vi "De-embed S-parameters - execute.vi"(4 "Truncate index":i32, 5 "Right info":T1, 6 "Truncate files":bool, 7 "Left info":T1, 8 "error in (no error)":errorcluster, 9 "Ignore lowest freq":bool caption="Ignore lowest frequency point (ISD discards it)", 10 "Horizontal Progress Bar":refnum<vi>, 11 "DUT+Fixture":path) -> (0 "error out":errorcluster)   [LabVIEW 2020]
uses:
  <vilib>/addons/HF Network Analysis/Support VIs/Read SnP File (SnP).vi
  <vilib>/addons/HF Network Analysis/NI_HFNetworkAnalysis.lvlib
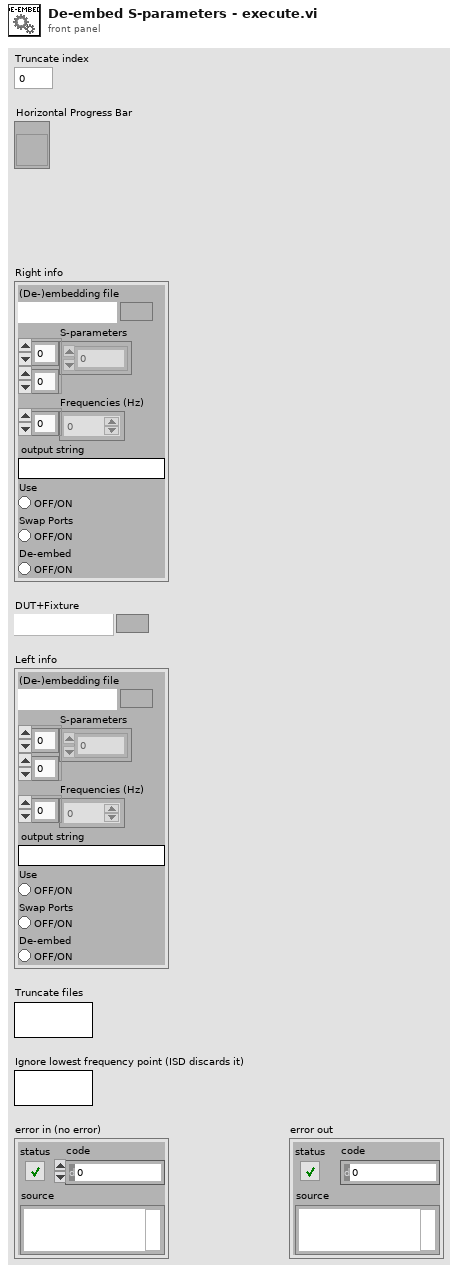
[diagram p1: front panel]
types:
  T1 = cluster{"(De-)embedding file":path, "S-parameters":cdb[][], "Frequencies (Hz)":dbl[], "output string":string, "Use":bool, "Swap Ports":bool, "De-embed":bool}
  T2 = enum16{"Check", "Read left", "Read right", "De-embed", "Exit"}
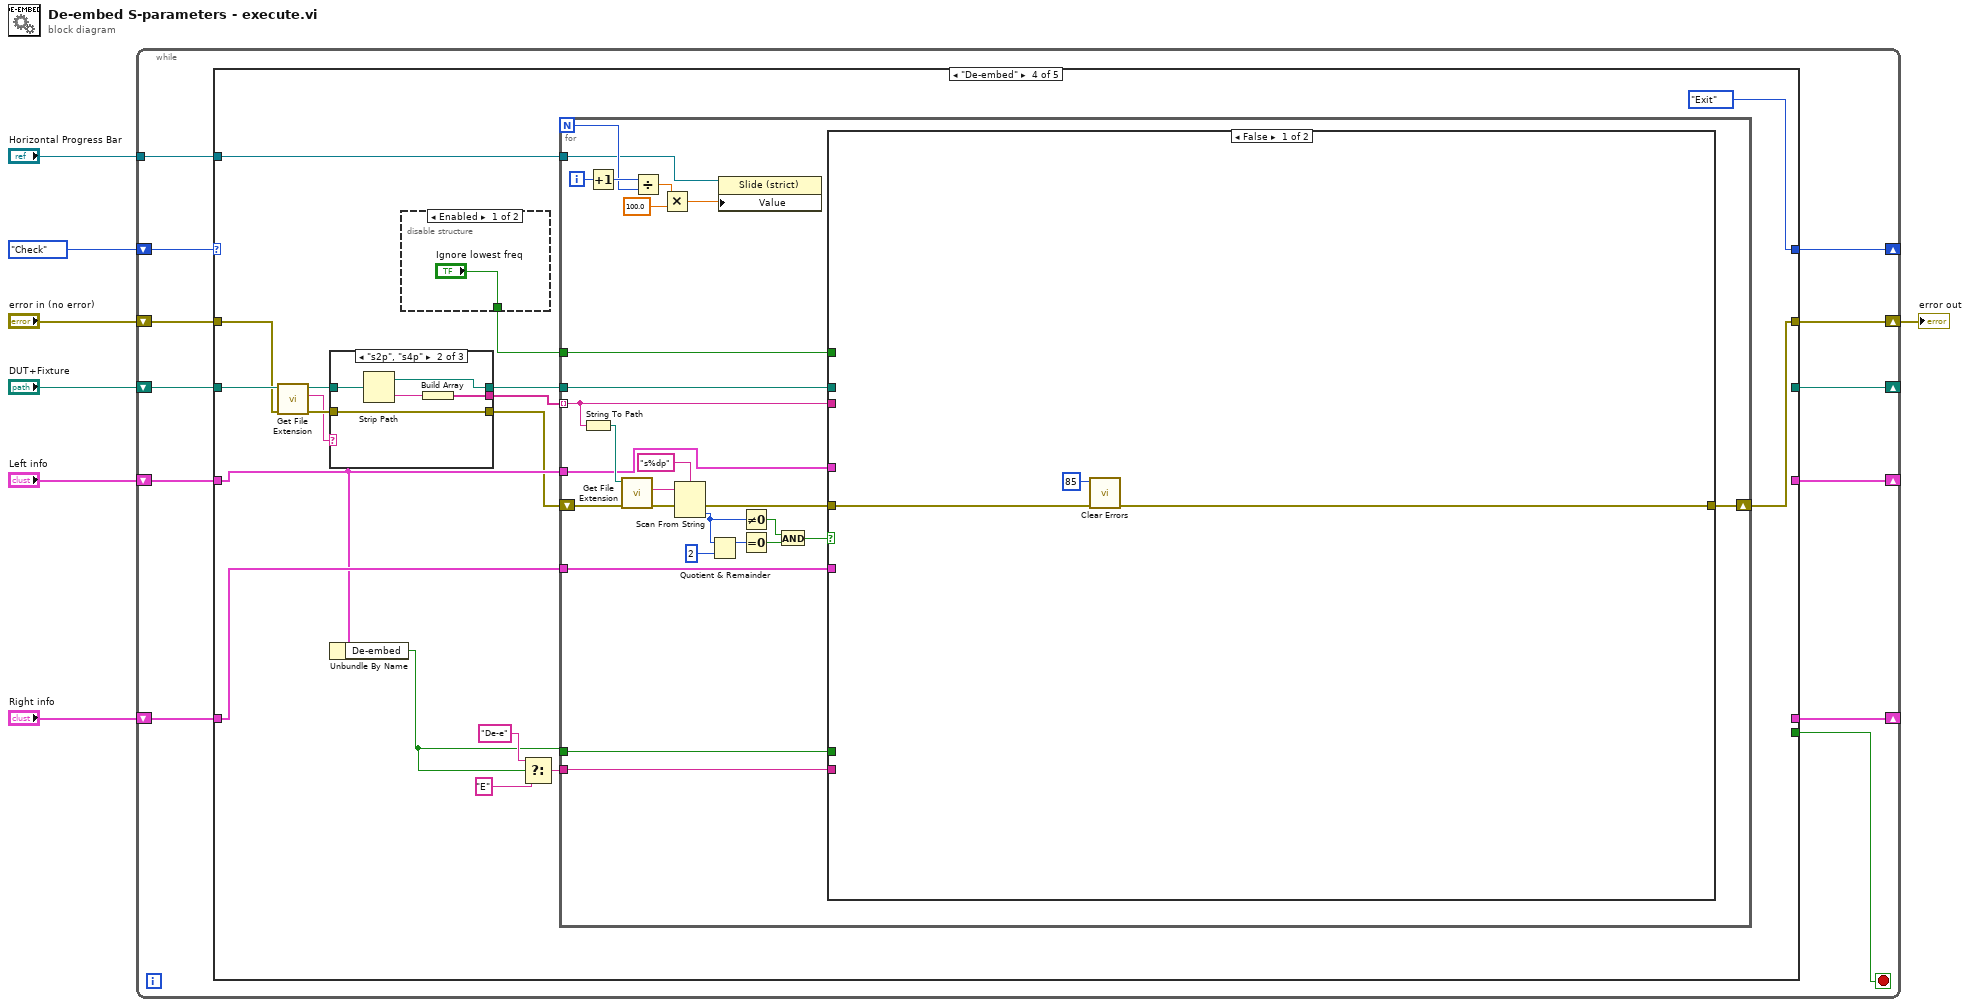
[diagram p0: block diagram]
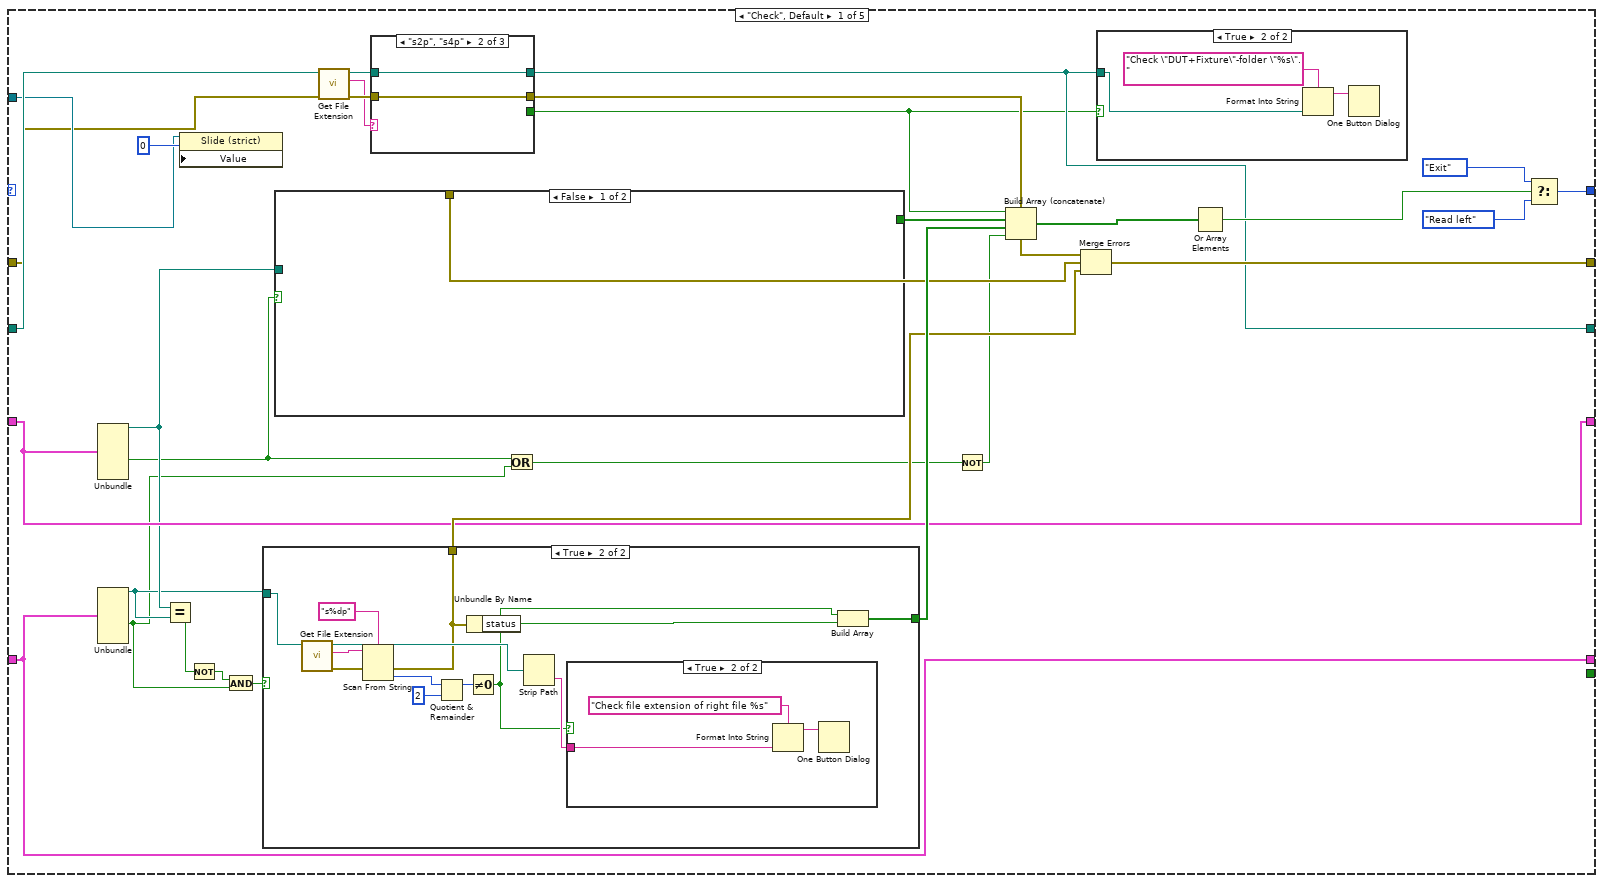
[diagram p2: hidden frame]
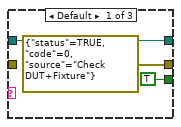
[diagram p3: hidden frame]
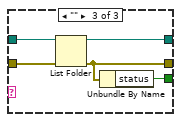
[diagram p4: hidden frame]
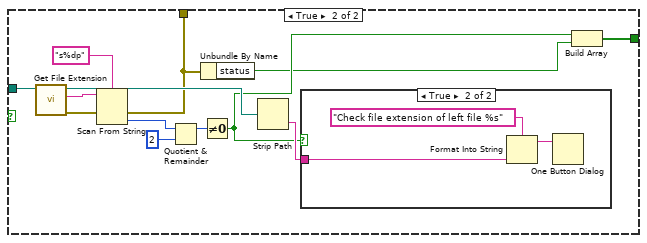
[diagram p6: hidden frame]
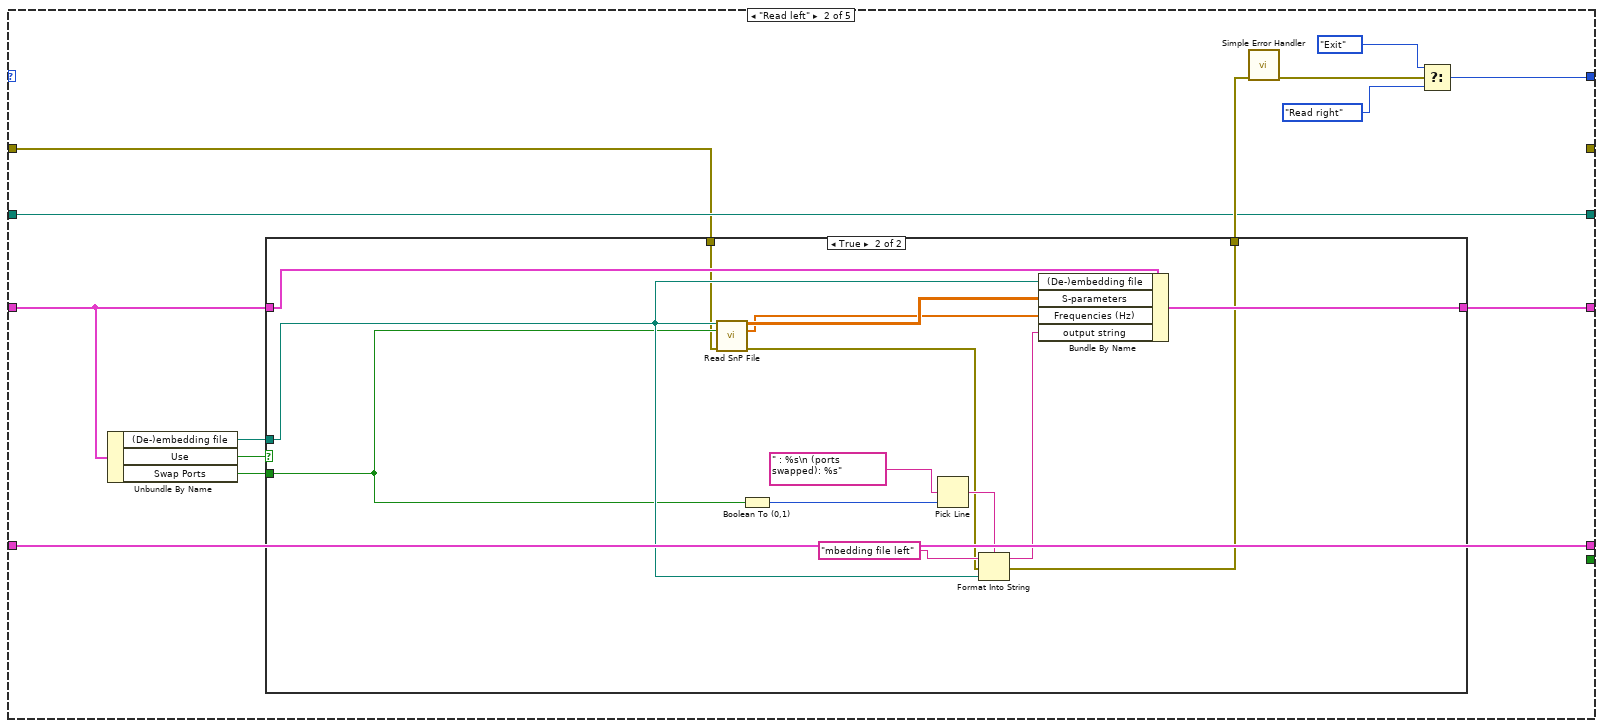
[diagram p10: hidden frame]
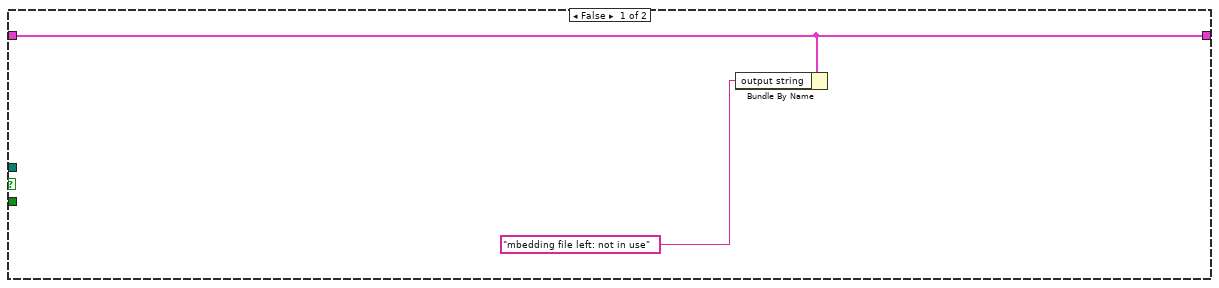
[diagram p11: hidden frame]
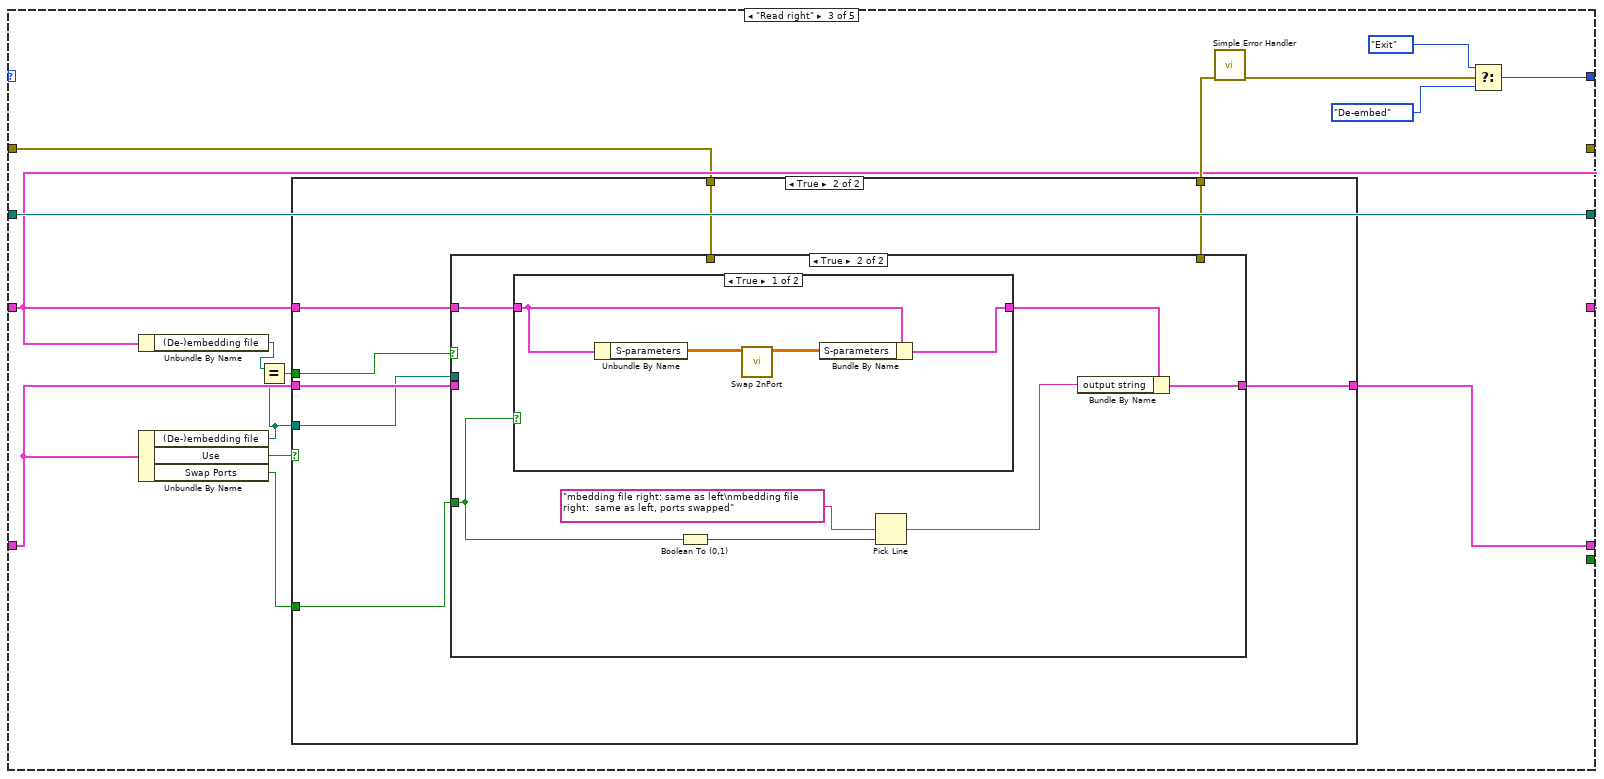
[diagram p12: hidden frame]
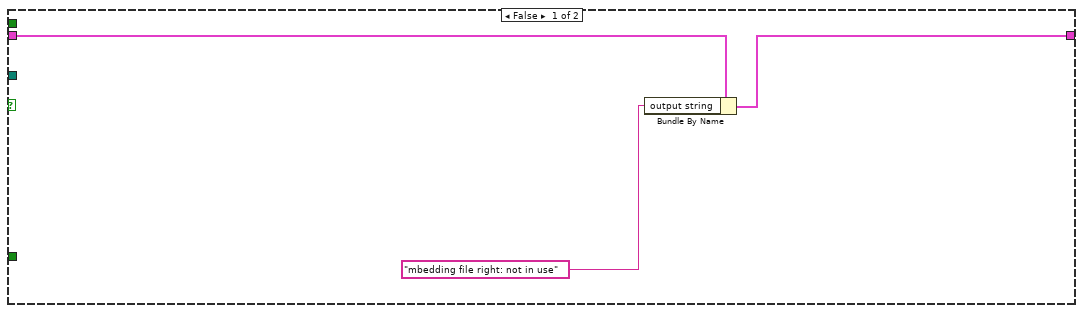
[diagram p13: hidden frame]
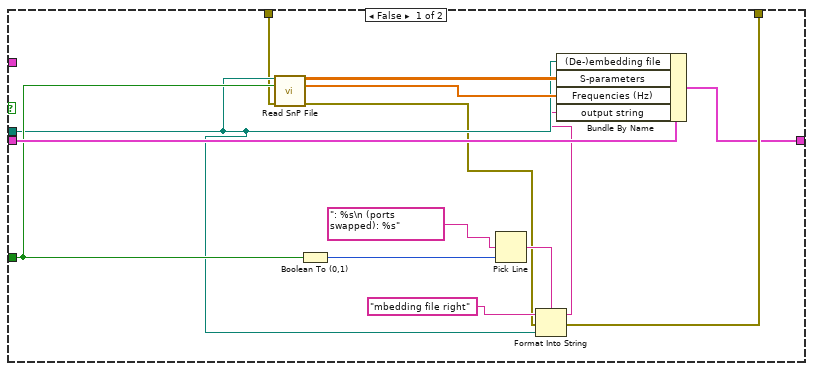
[diagram p14: hidden frame]
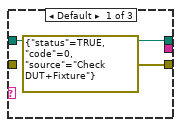
[diagram p17: hidden frame]
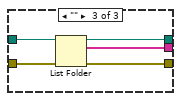
[diagram p18: hidden frame]
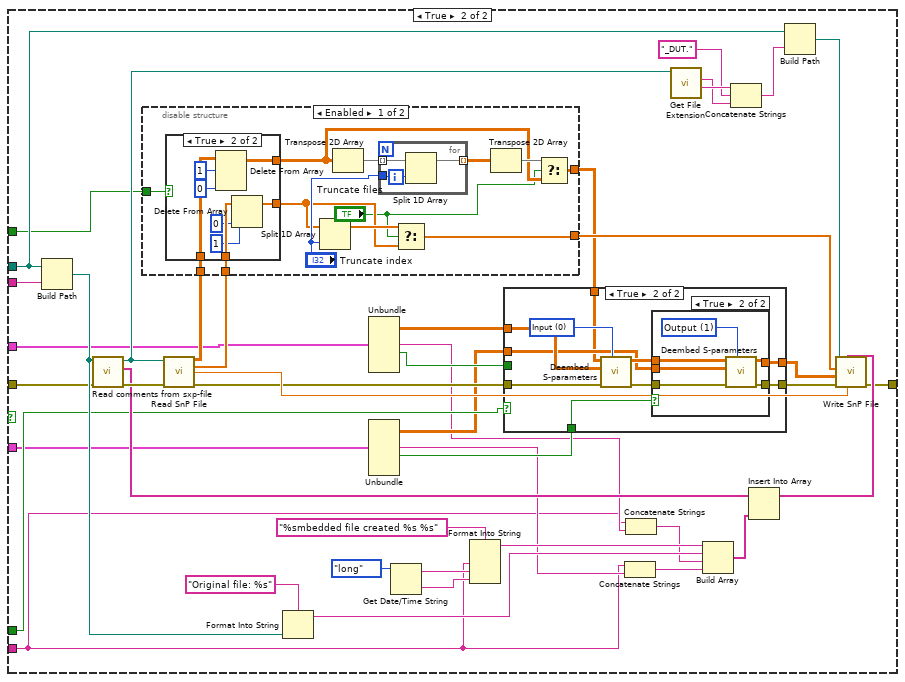
[diagram p19: hidden frame]
diagram:
  n1 = while {
    shift-right: [w16] -> _
    shift-left: "DUT+Fixture" -> [w18]
    shift-right: [w15] -> _
    shift-left: T2."Check" -> [w19]
    shift-right: [w14] -> _
    shift-left: "Left info" -> [w12]
    shift-right: [w13] -> _
    shift-left: "Right info" -> [w11]
    shift-right: [w10] -> w3
    shift-left: "error in (no error)" -> [w9]
    tunnel: "Horizontal Progress Bar" -> [w8]
    stop <- w17 stop-if-true
    n2 = case shown="\"De-embed\"" w19 {
      tunnel: w11 -> [w35 w103 w132 w189 w352]
      tunnel: w12 -> [w36 w100 w130 w188 w353]
      tunnel: w18 -> [w31 w102 w134 w182 _]
      tunnel: [_ _ _ _ TRUE] -> w17
      tunnel: [w22 w102 w134 _ path "" ("path out")] -> w16
      tunnel: [w46 w106 w137 T2."Exit" T2."Check"] -> w15
      tunnel: [w36 w101 w130 _ w353] -> w14
      tunnel: [w35 w103 w133 _ w352] -> w13
      tunnel: [w37 _ _ w179 w351] -> w10
      tunnel: w9 -> [w21 w96 w125 w178 w351]
      tunnel: w8 -> [w27 _ _ w186 _]
      frame "Check", Default {
        n3 = Unbundle(w36) -> ("(De-)embedding file"=w34:path, "Use"=w26:bool)  [unwired: 5 out]
        n4 = Unbundle(w35) -> ("(De-)embedding file"=w33:path, "Use"=w25:bool)  [unwired: 5 out]
        n5 = Equal?(x=w34, y=w33) -> (x = y?=w32:bool)
        n6 = property class="Slide (strict)"(reference=w27, "Value"=u8 0 ("Horizontal Progress Bar")) -> ()  [unwired: 1 in, 2 out]
        n7 = Not(x=w32) -> (.not. x?=w43:bool)
        n8 = And(x=w43, y=w25) -> (x .and. y?=w42:bool)
        n9 = case shown="True" w42 {
          tunnel: w33 -> [_ w85]
          tunnel: [_ w81] -> w44
          tunnel: [_ w80] -> w38
          frame False {
          }
          frame True {
            n10 = call <vilib>:"Get File Extension.vi"("file"=w85) -> ("error out"=w88:errorcluster, "lowercase file extension"=w86:string, "dup file"=w84:path)  [unwired: 6 in, 2 out]
            n11 = Scan From String(format string="s%dp", input string=w86, error in=w88) -> (error out=w80:errorcluster, output 1=w91:i32)  [unwired: 2 in, 2 out]
            n12 = Quotient & Remainder(x=w91, y=2) -> (x-y*floor(x/y)=w90:i32)  [unwired: 1 out]
            n13 = Unbundle By Name(w80) -> ("status"=w82:bool)
            n14 = Not Equal To 0?(x=w90) -> (x != 0?=w83:bool)
            n15 = Strip Path(path=w84) -> (name=w92:string)  [unwired: 1 out]
            n16 = case shown="True" w83 {
              tunnel: w92 -> [_ w93]
              frame False {
              }
              frame True {
                n17 = Format Into String(format string="Check file extension of right file %s", w93) -> (resulting string=w94:string)  [unwired: 2 in, 1 out]
                n18 = One Button Dialog(message=w94) -> ()  [unwired: 1 in, 1 out]
              }
            }
            n19 = Build Array(w83, w82) -> (w81:bool[])
          }
        }
        n20 = case shown="False" w26 {
          tunnel: [_ w65] -> w45
          tunnel: w34 -> [_ w69]
          tunnel: [_ w64] -> w39
          frame False {
          }
          frame True {
            n21 = call <vilib>:"Get File Extension.vi"("file"=w69) -> ("error out"=w74:errorcluster, "lowercase file extension"=w76:string, "dup file"=w68:path)  [unwired: 6 in, 2 out]
            n22 = Scan From String(format string="s%dp", input string=w76, error in=w74) -> (error out=w64:errorcluster, output 1=w71:i32)  [unwired: 2 in, 2 out]
            n23 = Quotient & Remainder(x=w71, y=2) -> (x-y*floor(x/y)=w72:i32)  [unwired: 1 out]
            n24 = Unbundle By Name(w64) -> ("status"=w66:bool)
            n25 = Not Equal To 0?(x=w72) -> (x != 0?=w67:bool)
            n26 = Strip Path(path=w68) -> (name=w70:string)  [unwired: 1 out]
            n27 = case shown="True" w67 {
              tunnel: w70 -> [_ w77]
              frame False {
              }
              frame True {
                n28 = Format Into String(format string="Check file extension of left file %s", w77) -> (resulting string=w78:string)  [unwired: 2 in, 1 out]
                n29 = One Button Dialog(message=w78) -> ()  [unwired: 1 in, 1 out]
              }
            }
            n30 = Build Array(w67, w66) -> (w65:bool[])
          }
        }
        n31 = call <vilib>:"Get File Extension.vi"("error in (no error)"=w21, "file"=w31) -> ("error out"=w29:errorcluster, "lowercase file extension"=w28:string, "dup file"=w30:path)  [unwired: 5 in, 2 out]
        n32 = case shown="\"s2p\", \"s4p\"" w28 {
          tunnel: [errorcluster {"status"=TRUE, "code"=0, "source"="Check DUT+Fixture"} ("error out") w55 w60] -> w40
          tunnel: [w53 w54 w59] -> w22
          tunnel: w30 -> [w53 w54 w58]
          tunnel: w29 -> [_ w55 w57]
          tunnel: [TRUE ("status") _ w56] -> w20
          frame Default {
          }
          frame "s2p", "s4p" {
          }
          frame "" {
            n33 = List Folder(path=w58, error in=w57) -> (path out=w59:path, error out=w60:errorcluster)  [unwired: 2 in, 2 out]
            n34 = Unbundle By Name(w60) -> ("status"=w56:bool)
          }
        }
        n35 = Or(x=w26, y=w25) -> (x .or. y?=w24:bool)
        n36 = Not(x=w24) -> (.not. x?=w23:bool)
        n37 = Build Array (concatenate)(w20, w45, w44, w23) -> (w50:bool[])
        n38 = Merge Errors(w40, w39, w38) -> (w37:errorcluster)
        n39 = case shown="True" w20 {
          tunnel: w22 -> [_ w61]
          frame False {
          }
          frame True {
            n40 = Format Into String(format string="Check \"DUT+Fixture\"-folder \"%s\".", w61) -> (resulting string=w62:string)  [unwired: 2 in, 1 out]
            n41 = One Button Dialog(message=w62) -> ()  [unwired: 1 in, 1 out]
          }
        }
        n42 = Or Array Elements(Boolean array=w50) -> (logical OR=w47:bool)
        n43 = Select(t=T2."Exit", s=w47, f=T2."Read left") -> (s? t:f=w46:T2)
      }
      frame "Read left" {
        n44 = Unbundle By Name(w100) -> ("(De-)embedding file"=w98:path, "Use"=w99:bool, "Swap Ports"=w97:bool)
        n45 = case shown="True" w99 {
          tunnel: [_ w113] -> w105
          tunnel: [w110 w120] -> w101
          tunnel: w100 -> [w110 w119]
          tunnel: w98 -> [_ w117]
          tunnel: w97 -> [_ w112]
          tunnel: w96 -> [_ w111]
          frame False {
            n46 = Bundle By Name(cluster=w110, "output string"="mbedding file left: not in use" ("format string")) -> ()  [unwired: 1 out]
          }
          frame True {
            n47 = call-poly <vilib>:"Read SnP File.vi"("SnP File Path"=w117, "Swap Ports (False)"=w112, "Error In"=w111) -> ("S-parameters"=w124:cdb[][], "Frequencies (Hz)"=w123:dbl[], "Error Out"=w114:errorcluster)  [unwired: 9 in, 1 out]
            n48 = Boolean To (0,1)(Boolean=w112) -> (0, 1=w122:i16)
            n49 = Pick Line(multi-line string=" : %s\n (ports swapped): %s" ("format string"), line index=w122) -> (output string=w116:string)  [unwired: 1 in]
            n50 = Format Into String(format string=w116, initial string="mbedding file left" ("format string"), error in=w114, w117) -> (resulting string=w115:string, error out=w113:errorcluster)
            n51 = Bundle By Name(cluster=w119, "(De-)embedding file"=w117, "S-parameters"=w124, "Frequencies (Hz)"=w123, "output string"=w115) -> (w120:T1)
          }
        }
        n52 = call <vilib>:"Simple Error Handler.vi"("error in (no error)"=w105) -> ("error out"=w104:errorcluster)  [unwired: 4 in, 4 out]
        n53 = Select(t=T2."Exit", s=w104, f=T2."Read right") -> (s? t:f=w106:T2)
      }
      frame "Read right" {
        n54 = Unbundle By Name(w130) -> ("(De-)embedding file"=w129:path)
        n55 = Unbundle By Name(w132) -> ("(De-)embedding file"=w128:path, "Use"=w131:bool, "Swap Ports"=w126:bool)
        n56 = Equal?(x=w129, y=w128) -> (x = y?=w127:bool)
        n57 = case shown="True" w131 {
          tunnel: [_ w150] -> w136
          tunnel: [w140 w143] -> w133
          tunnel: w130 -> [_ w144]
          tunnel: w132 -> [w141 w149]
          tunnel: w128 -> [_ w148]
          tunnel: w127 -> [_ w147]
          tunnel: w126 -> [_ w146]
          tunnel: w125 -> [_ w145]
          frame False {
            n58 = Bundle By Name(cluster=w141, "output string"="mbedding file right: not in use" ("format string")) -> (w140:T1)
          }
          frame True {
            n59 = case shown="True" w147 {
              tunnel: [w154 _] -> w150
              tunnel: w148 -> [w158 _]
              tunnel: w149 -> [w162 _]
              tunnel: w146 -> [w161 w167]
              tunnel: w145 -> [w152 _]
              tunnel: w144 -> [_ w166]
              tunnel: [w151 w168] -> w143
              frame False {
                n60 = call-poly <vilib>:"Read SnP File.vi"("SnP File Path"=w158, "Swap Ports (False)"=w161, "Error In"=w152) -> ("S-parameters"=w164:cdb[][], "Frequencies (Hz)"=w163:dbl[], "Error Out"=w155:errorcluster)  [unwired: 9 in, 1 out]
                n61 = Boolean To (0,1)(Boolean=w161) -> (0, 1=w153:i16)
                n62 = Pick Line(multi-line string=": %s\n (ports swapped): %s" ("format string"), line index=w153) -> (output string=w157:string)  [unwired: 1 in]
                n63 = Format Into String(format string=w157, initial string="mbedding file right" ("format string"), error in=w155, w158) -> (resulting string=w156:string, error out=w154:errorcluster)
                n64 = Bundle By Name(cluster=w162, "(De-)embedding file"=w158, "S-parameters"=w164, "Frequencies (Hz)"=w163, "output string"=w156) -> (w151:T1)
              }
              frame True {
                n65 = case shown="True" w167 {
                  tunnel: w166 -> [w174 w176]
                  tunnel: [w175 w176] -> w165
                  frame True {
                    n66 = Unbundle By Name(w174) -> ("S-parameters"=w173:cdb[][])
                    n67 = call <vilib>:"Swap 2nPort.vi"("Parameters In (2D)"=w173) -> ("Parameters Out (2D)"=w172:cdb[][])  [unwired: 9 in, 1 out]
                    n68 = Bundle By Name(cluster=w174, "S-parameters"=w172) -> (w175:T1)
                  }
                  frame False {
                  }
                }
                n69 = Boolean To (0,1)(Boolean=w167) -> (0, 1=w171:i16)
                n70 = Pick Line(multi-line string="mbedding file right: same as left\nmbedding file right:  same as left, ports swapped" ("format string"), line index=w171) -> (output string=w169:string)  [unwired: 1 in]
                n71 = Bundle By Name(cluster=w165, "output string"=w169) -> (w168:T1)
              }
            }
          }
        }
        n72 = call <vilib>:"Simple Error Handler.vi"("error in (no error)"=w136) -> ("error out"=w135:errorcluster)  [unwired: 4 in, 4 out]
        n73 = Select(t=T2."Exit", s=w135, f=T2."De-embed") -> (s? t:f=w137:T2)
      }
      frame "De-embed" {
        n74 = call <vilib>:"Get File Extension.vi"("error in (no error)"=w178, "file"=w182) -> ("error out"=w184:errorcluster, "lowercase file extension"=w183:string, "dup file"=w185:path)  [unwired: 5 in, 2 out]
        n75 = case shown="\"s2p\", \"s4p\"" w183 {
          tunnel: [errorcluster {"status"=TRUE, "code"=0, "source"="Check DUT+Fixture"} ("error out") w202 w207] -> w177
          tunnel: [w197 w200 w206] -> w181
          tunnel: w185 -> [w197 w201 w205]
          tunnel: w184 -> [_ w202 w204]
          tunnel: [_ w198 w203] -> w180
          frame Default {
          }
          frame "s2p", "s4p" {
            n76 = Strip Path(path=w201) -> (stripped path=w200:path, name=w199:string)
            n77 = Build Array(w199) -> (w198:string[])
          }
          frame "" {
            n78 = List Folder(path=w205, error in=w204) -> (path out=w206:path, filenames=w203:string[], error out=w207:errorcluster)  [unwired: 2 in, 1 out]
          }
        }
        n79 = Unbundle By Name(w188) -> ("De-embed"=w187:bool)
        n80 = disable-structure shown="Enabled" {
          disable-tunnel: ["Ignore lowest freq" _] -> w194
          frame Enabled {
          }
          frame Disabled {
          }
        }
        n81 = Select(t="De-e" ("format string"), s=w187, f="E" ("format string")) -> (s? t:f=w191:string)
        n82 = for {
          N -> [w212]
          tunnel: w181 -> [w234]
          tunnel: w180 -> [w233] mode=indexing
          tunnel: w194 -> [w229]
          tunnel: w191 -> [w228]
          tunnel: w187 -> [w227]
          tunnel: w188 -> [w216]
          tunnel: w189 -> [w215]
          tunnel: w186 -> [w211]
          shift-right: [w209] -> w179
          shift-left: w177 -> [w208]
          i -> [w231]
          n83 = String To Path(string=w233) -> (path=w232:path)
          n84 = Increment(x=w231) -> (x+1=w230:i32)
          n85 = call <vilib>:"Get File Extension.vi"("error in (no error)"=w208, "file"=w232) -> ("error out"=w226:errorcluster, "lowercase file extension"=w224:string)  [unwired: 5 in, 3 out]
          n86 = Divide(x=w230, y=w212) -> (x/y=w214:dbl)
          n87 = Multiply(x=w214, y=100.0) -> (x*y=w210:dbl)
          n88 = Scan From String(format string="s%dp", input string=w224, error in=w226) -> (error out=w225:errorcluster, output 1=w218:i32)  [unwired: 2 in, 2 out]
          n89 = Quotient & Remainder(x=w218, y=2) -> (x-y*floor(x/y)=w222:i32)  [unwired: 1 out]
          n90 = property class="Slide (strict)"(reference=w211, "Value"=w210) -> ()  [unwired: 1 in, 2 out]
          n91 = Not Equal To 0?(x=w218) -> (x != 0?=w217:bool)
          n92 = Equal To 0?(x=w222) -> (x = 0?=w220:bool)
          n93 = And(x=w217, y=w220) -> (x .and. y?=w219:bool)
          n94 = case shown="False" w219 {
            tunnel: w233 -> [_ w272]
            tunnel: w234 -> [_ w261]
            tunnel: w225 -> [w237 w258]
            tunnel: w229 -> [_ w253]
            tunnel: w228 -> [_ w239]
            tunnel: w227 -> [_ w250]
            tunnel: w216 -> [_ w249]
            tunnel: w215 -> [_ w246]
            tunnel: [w236 w238] -> w209
            frame False {
              n95 = call <vilib>:"Clear Errors.vi"("error in (no error)"=w237, "specific error code to clear (0: all)"=85) -> ("error out"=w236:errorcluster)  [unwired: 4 in, 1 out]
            }
            frame True {
              n96 = Build Path(base path=w261, name or relative path=w272) -> (appended path=w260:path)
              n97 = call "Read comments from sxp-file.vi"("error in (no error)"=w258, "file path"=w260) -> ("error out"=w257:errorcluster, "Comment lines"=w254:string[], "file path out"=w259:path)  [unwired: 7 in]
              n98 = call-poly <vilib>:"Read SnP File.vi"("SnP File Path"=w259, "Error In"=w257) -> ("S-parameters"=w264:cdb[][], "Frequencies (Hz)"=w263:dbl[], "Z0 (Ohm)"=w280:cdb, "Error Out"=w262:errorcluster)  [unwired: 10 in]
              n99 = disable-structure shown="Enabled" {
                disable-tunnel: w264 -> [w293 w308]
                disable-tunnel: w263 -> [w292 w307]
                disable-tunnel: w253 -> [w291 _]
                disable-tunnel: [w285 w307] -> w252
                disable-tunnel: [w283 w308] -> w251
                frame Enabled {
                  n100 = case shown="True" w291 {
                    tunnel: w293 -> [w297 w306]
                    tunnel: [w297 w305] -> w282
                    tunnel: w292 -> [w298 w304]
                    tunnel: [w298 w303] -> w286
                    frame False {
                    }
                    frame True {
                      n101 = Delete From Array(array=w306, length=1, index (row)=0) -> (array with subset deleted=w305:cdb[][])  [unwired: 1 in, 1 out]
                      n102 = Delete From Array(array=w304, length=1, index=0) -> (array with subset deleted=w303:dbl[])  [unwired: 1 out]
                    }
                  }
                  n103 = Split 1D Array(array=w286, index="Truncate index") -> (first subarray=w287:dbl[])  [unwired: 1 out]
                  n104 = Transpose 2D Array(2D array=w282) -> (transposed array=w288:cdb[][])
                  n105 = for {
                    tunnel: [w296] -> w289 mode=indexing
                    tunnel: "Truncate index" -> [w295]
                    tunnel: w288 -> [w294] mode=indexing
                    n106 = Split 1D Array(array=w294, index=w295) -> (first subarray=w296:cdb[])  [unwired: 1 out]
                  }
                  n107 = Select(t=w287, s="Truncate files", f=w286) -> (s? t:f=w285:dbl[])
                  n108 = Transpose 2D Array(2D array=w289) -> (transposed array=w284:cdb[][])
                  n109 = Select(t=w284, s="Truncate files", f=w282) -> (s? t:f=w283:cdb[][])
                }
                frame Disabled {
                }
              }
              n110 = Format Into String(format string="Original file: %s", w260) -> (resulting string=w265:string)  [unwired: 2 in, 1 out]
              n111 = Unbundle(w249) -> ("S-parameters"=w248:cdb[][], "output string"=w243:string, "Use"=w247:bool)  [unwired: 4 out]
              n112 = Unbundle(w246) -> ("S-parameters"=w245:cdb[][], "output string"=w241:string, "Use"=w244:bool)  [unwired: 4 out]
              n113 = Get Date/Time String(date format (0)=enum16{"short", "long", "abbreviated"}."long") -> (date string=w269:string, time string=w268:string)  [unwired: 2 in]
              n114 = Format Into String(format string="%smbedded file created %s %s", w239, w269, w268) -> (resulting string=w267:string)  [unwired: 2 in, 1 out]
              n115 = case shown="True" w250 {
                tunnel: [w311 w340] -> w279
                tunnel: [w312 w339] -> w278
                tunnel: w248 -> [w318 w338]
                tunnel: w245 -> [w314 w337]
                tunnel: w262 -> [w317 w336]
                tunnel: w251 -> [w315 w334]
                tunnel: w244 -> [w310 w333]
                tunnel: w247 -> [w309 _]
                frame False {
                  n116 = case shown="True" w309 {
                    tunnel: w318 -> [_ w332]
                    tunnel: w317 -> [w327 w331]
                    tunnel: [w326 w330] -> w316
                    tunnel: w315 -> [w326 w329]
                    tunnel: [w327 w328] -> w313
                    frame False {
                    }
                    frame True {
                      n117 = call <vilib>:"Cascade S-parameters.vi"("error in (no error)"=w331, "S-par array 2 in"=w329, "S-par array 1 in"=w332) -> ("error out"=w328:errorcluster, "Cascaded S-par array out"=w330:cdb[][])  [unwired: 7 in]
                    }
                  }
                  n118 = case shown="True" w310 {
                    tunnel: w316 -> [w320 w325]
                    tunnel: w314 -> [_ w324]
                    tunnel: w313 -> [w319 w323]
                    tunnel: [w319 w322] -> w312
                    tunnel: [w320 w321] -> w311
                    frame False {
                    }
                    frame True {
                      n119 = call <vilib>:"Cascade S-parameters.vi"("error in (no error)"=w323, "S-par array 2 in"=w324, "S-par array 1 in"=w325) -> ("error out"=w322:errorcluster, "Cascaded S-par array out"=w321:cdb[][])  [unwired: 7 in]
                    }
                  }
                }
                frame True {
                  w342 = u16 0 items=["Input", "Output"] ("Deembedding Side")
                  n120 = call <vilib>:"Deembed S-parameters.vi"("Deembedding Side"=w342, "error in (no error)"=w336, "Deembedding S-par array in"=w338, "Original S-par array in"=w334) -> ("error out"=w335:errorcluster, "Deembedded S-par array out"=w341:cdb[][])  [unwired: 6 in]
                  n121 = case shown="True" w333 {
                    tunnel: w341 -> [w343 w350]
                    tunnel: [w343 w348] -> w340
                    tunnel: [w344 w347] -> w339
                    tunnel: w337 -> [_ w346]
                    tunnel: w335 -> [w344 w345]
                    frame False {
                    }
                    frame True {
                      w349 = u16 1 items=["Input", "Output"] ("Deembedding Side")
                      n122 = call <vilib>:"Deembed S-parameters.vi"("Deembedding Side"=w349, "error in (no error)"=w345, "Deembedding S-par array in"=w346, "Original S-par array in"=w350) -> ("error out"=w347:errorcluster, "Deembedded S-par array out"=w348:cdb[][])  [unwired: 6 in]
                    }
                  }
                }
              }
              n123 = Concatenate Strings(w239, w241) -> (w240:string)
              n124 = Concatenate Strings(w239, w243) -> (w242:string)
              n125 = call <vilib>:"Get File Extension.vi"("file"=w259) -> ("filename without extension"=w277:string, "lowercase file extension"=w275:string)  [unwired: 6 in, 3 out]
              n126 = Build Array(w267, w265, w242, w240) -> (w256:string[])
              n127 = Concatenate Strings(w277, "_DUT." ("string"), w275) -> (w274:string)
              n128 = Insert Into Array(array=w254, new element=w256) -> (w255:string[])  [unwired: 1 in]
              n129 = Build Path(base path=w261, name or relative path=w274) -> (appended path=w273:path)
              n130 = call <vilib>:"Write SnP File.vi"("Z0 (50 Ohm)"=w280, "Comments"=w255, "error in (no error)"=w278, "S-parameters"=w279, "Frequencies (Hz)"=w252, "SnP File Path"=w273) -> ("error out"=w238:errorcluster)  [unwired: 5 in]
            }
          }
        }
      }
      frame "Exit" {
      }
    }
  }
  "error out" <- w3
